vi "Read Module Menu Name.vi"(8 "error in":errorcluster, 11 "Watchdog editor node in":refnum<class "Watchdog editor node.lvclass">) -> (0 "error out":errorcluster, 2 "Menu Name":string, 3 "Watchdog editor node out":refnum<class "Watchdog editor node.lvclass">)   [LabVIEW 2013, in "Watchdog editor node.lvclass"]
uses:
  Watchdog editor node.lvclass
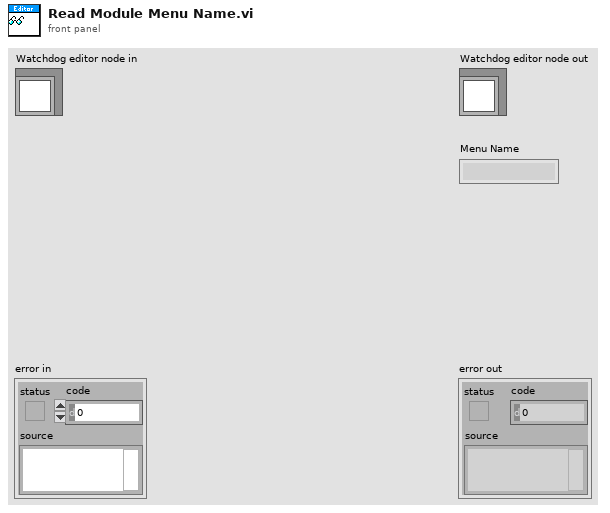
[diagram p1: front panel]
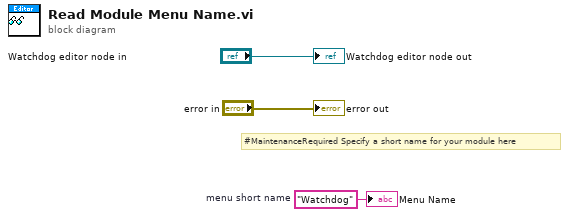
[diagram p0: block diagram]
diagram:
  w1 = "Watchdog"  # menu short name
  # "#MaintenanceRequired Specify a short name for your module here"
  "error out" <- "error in"
  "Watchdog editor node out" <- "Watchdog editor node in"
  "Menu Name" <- w1
